vi "SigProc_subVI makingKernel.vi"(7 "Type":u8=1 min=1, 8 "error in (no error)":errorcluster, 10 "dt":dbl, 11 "Window":dbl=1.0 min=1.0 max=100000.0) -> (0 "error out":errorcluster, 2 "kernel":sgl[](array[numeric]), 3 "window":i32)   [LabVIEW 2018, in "Sig2MS.lvclass"]
uses:
  Sig2MS.lvclass
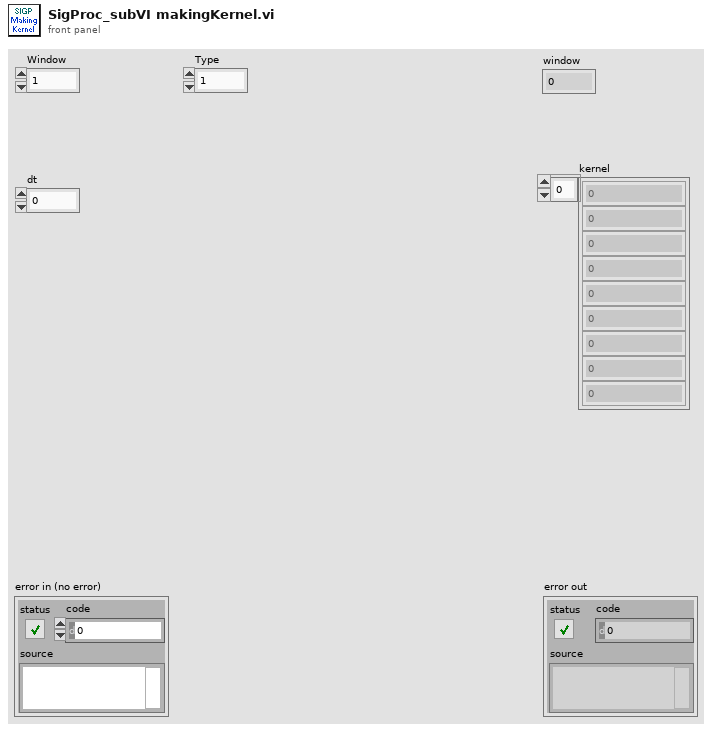
[diagram p1: front panel]
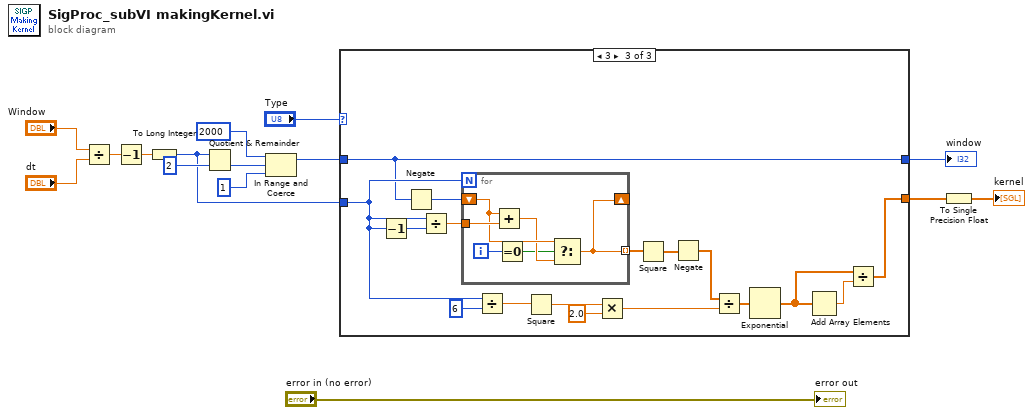
[diagram p0: block diagram]
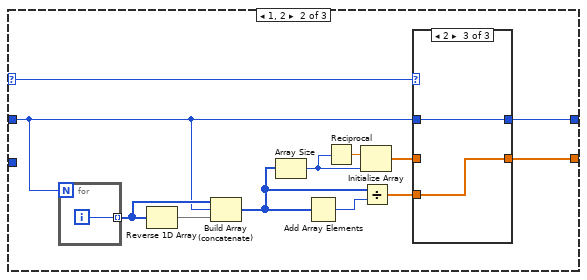
[diagram p3: hidden frame]
diagram:
  n1 = Divide(x="Window", y="dt") -> (x/y=w13:dbl)
  n2 = Decrement(x=w13) -> (x-1=w11:dbl)
  n3 = To Long Integer(number=w11) -> (32bit integer=w7:i32)
  n4 = Quotient & Remainder(x=w7, y=2) -> (floor(x/y)=w9:i32)  [unwired: 1 out]
  n5 = In Range and Coerce(upper limit=2000, x=w9, lower limit=1) -> (coerced(x)=w8:i32)  [unwired: 1 out]
  n6 = case "Making kernel" shown="3" "Type" {
    selector: "Type" -> [_ w21 _]
    tunnel: w8 -> [_ w17 w35]
    tunnel: [_ w18 w36] -> w2
    tunnel: w7 -> [_ _ w39]
    tunnel: [_ w16 w35] -> w3
    frame 0, Default {
    }
    frame 1, 2 {
      n7 = for {
        N: w17 -> [_]
        tunnel: [w34] -> w26 mode=indexing
        i -> [w34]
      }
      n8 = Reverse 1D Array(array=w26) -> (reversed array=w27:i32[])
      n9 = Build Array (concatenate)(w26, w17, w27) -> (w24:i32[])
      n10 = Array Size(array=w24) -> (size(s)=w22:i32)
      n11 = Add Array Elements(numeric array=w24) -> (sum=w25:i32)
      n12 = Reciprocal(x=w22) -> (1/x=w23:dbl)
      n13 = Initialize Array(w23, w22) -> (w20:dbl[])
      n14 = Divide(x=w24, y=w25) -> (x/y=w19:dbl[])
      n15 = case shown="2" w21 {
        tunnel: w20 -> [w29 w30 _]
        tunnel: w19 -> [_ _ w32]
        tunnel: [w29 w30 w32] -> w18
        tunnel: w17 -> [w28 w31 w33]
        tunnel: [w28 w31 w33] -> w16
        frame 0, Default {
        }
        frame 1 {
        }
        frame 2 {
        }
      }
    }
    frame 3 {
      n16 = Decrement(x=w39) -> (x-1=w49:i32)
      n17 = Negate(x=w35) -> (-x=w50:i32)
      n18 = Divide(x=w39, y=w49) -> (x/y=w51:dbl)
      n19 = for {
        N: w39 -> [_]
        tunnel: w51 -> [w57]
        shift-right: [w54] -> _
        shift-left: w50 -> [w56]
        tunnel: [w54] -> w48 mode=indexing
        i -> [w53]
        n20 = Add(x=w56, y=w57) -> (x+y=w55:dbl)
        n21 = Equal To 0?(x=w53) -> (x = 0?=w52:bool)
        n22 = Select(t=w56, s=w52, f=w55) -> (s? t:f=w54:dbl)
      }
      n23 = Divide(x=w39, y=6) -> (x/y=w46:dbl)
      n24 = Square(x=w46) -> (x^2=w45:dbl)
      n25 = Multiply(x=w45, y=2.0) -> (x*y=w43:dbl)
      n26 = Square(x=w48) -> (x^2=w38:dbl[])
      n27 = Negate(x=w38) -> (-x=w37:dbl[])
      n28 = Divide(x=w37, y=w43) -> (x/y=w42:dbl[])
      n29 = Exponential(1:w42) -> (0:w40:dbl[])
      n30 = Add Array Elements(numeric array=w40) -> (sum=w41:dbl)
      n31 = Divide(x=w40, y=w41) -> (x/y=w36:dbl[])
    }
  }
  "window" <- w3
  n32 = To Single Precision Float(number=w2) -> (single precision float=→"kernel":sgl[])
  "error out" <- "error in (no error)"
